vi "PH_Stepmotor_BaseClass.PC Set Axis Information.vi"(0 "i ref in":refnum<vi>, 1 "axis":i32=-1, 3 "Current Position (Steps)":i32, 4 "Axis Activity":T1, 5 "error in (no error)":errorcluster) -> (14 "i ref out":refnum<vi>, 19 "error out":errorcluster)   [LabVIEW 2014, in "PH_Stepmotor_BaseClass.lvlib"]
doc: "This VI stores in case of a change relevant information to own attributes and updates related DIM services."
uses:
  PH_Stepmotor_BaseClass.lvlib
  PH_Stepmotor_BaseClass.Axis Activity.ctl
  PH_Stepmotor_BaseClass.Axis Information.ctl
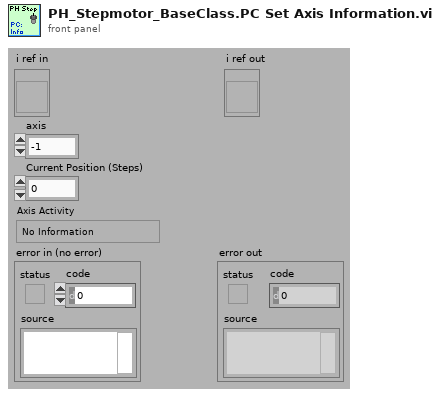
[diagram p1: front panel]
types:
  T1 = typedef "PH_Stepmotor_BaseClass.lvlib/PH_Stepmotor_BaseClass.Axis Activity.ctl" = enum16{"No Information", "stopped", "running", "Failure", "Alarm", "stopped at backward ES", "stopped at foreward ES"}
  T2 = typedef "PH_Stepmotor_BaseClass.lvlib/PH_Stepmotor_BaseClass.Axis Attributes.ctl" = cluster{"Settings":T3, "Endswitch?":bool, "DIM Service IDs":T5, "Activity":T1, "Configured?":bool, "Position":cluster{"Current":i32, "Target":i32}, "Position to set":cluster{"New?":bool, "Wanted":i32}, "Stop?":bool, "Reset?":bool, "Move?":bool, "Nothing connected?":bool}
  T3 = typedef "PH_Stepmotor_BaseClass.lvlib/PH_Stepmotor_BaseClass.Axis Settings.ctl" = cluster{"Sign change":bool, "Width":dbl, "Calibration":dbl, "Unit":string, "Motor Type":T4, "Unit Width":string, "Unit CF":string}
  T4 = typedef "PH_Stepmotor_BaseClass.lvlib/PH_Stepmotor_BaseClass.Motor Type.ctl" = enum16{"Unspecific", "OWIS 49.120.2633", "OWIS 49.060.1033", "OWIS 43.040.2558", "Diamond Motion 2200 series", "OWIS 49.120.266B.MV6", "Calorimeter", "Linear Stage 1", "MICOS VT-80", "MICOS VT-80 S", "Standa Rotstage nt0.95A", "PUF RA 320.200", "PUF RA 800.200", "PUF RA 800.400", "PUF RA 400.50", "1324.nn.800.50", "1324.n9c.800.50", "1324.nn.320.200", "1324.nn.400.200", "1324.nn.800.200", "1324.nn.400.50", "1324.8c9c.800.50", "1324.8c9c.400.200"}
  T5 = typedef "PH_Stepmotor_BaseClass.lvlib/PH_Stepmotor_BaseClass.Axis DIM Service IDs.ctl" = cluster{"Settings":i32, "Information":i32}
  T6 = typedef "PH_Stepmotor_BaseClass.lvlib/PH_Stepmotor_BaseClass.Axis Information.ctl" = cluster{"Scaled Position":dbl, "Activity":T1}
  T7 = typedef "PH_Stepmotor_BaseClass.lvlib/PH_Stepmotor_BaseClass.i attribute.ctl" = cluster{"Device Error":errorcluster, "Axes PSDB Thread":cluster{"Ref":refnum<vi>, "Q-Ref":refnum<queue>, "Data Status":T8}, "Axes":T2[], "Axes PSDB Infos":cluster{"GUI Name":string, "PSDB Instance ID":i32, "PSDB Status Service ID":i32, "Axis":i32, "Class":string}[], "GUI Refs":T9}
  T8 = typedef "PH_PSDBWriter.lvlib/PH_PSDBWriter.Data Status.ctl" = i16
  T9 = typedef "PH_Stepmotor_BaseClass.lvlib/PH_Stepmotor_BaseClass.GUI Refs.ctl" = cluster{"Axes Configuration":refnum<vi>, "Device Error":refnum<vi>, "Axes PSDB Infos":refnum<vi>}
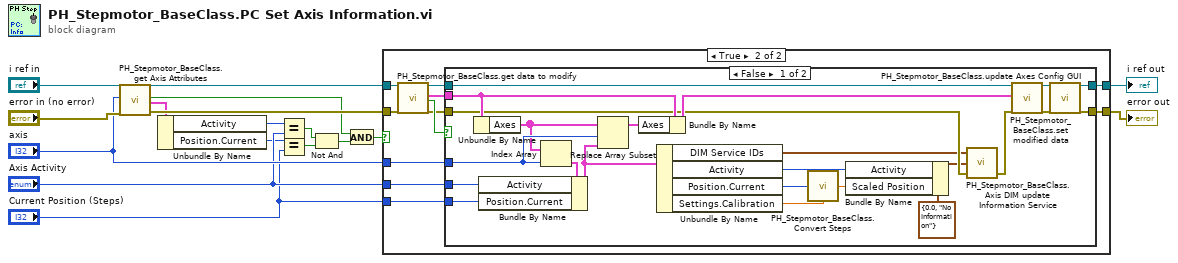
[diagram p0: block diagram]
diagram:
  n1 = call "PH_Stepmotor_BaseClass.get Axis Attributes.vi"("VI in"="i ref in", "Axis"="axis", "error in (no error)"="error in (no error)") -> ("VI out"=w12:refnum<vi>, "Axis found?"=w7:bool, "Axis Attributes"=w10:T2, "error out"=w14:errorcluster)  [unwired: 13 in]
  n2 = Unbundle By Name(w10) -> ("Activity"=w9:T1, "Position.Current"=w5:i32)
  n3 = Equal?(x=w9, y="Axis Activity") -> (x = y?=w3:bool)
  n4 = Equal?(x=w5, y="Current Position (Steps)") -> (x = y?=w2:bool)
  n5 = Not And(1:w2, 2:w3) -> (0:w1:bool)
  n6 = And(x=w7, y=w1) -> (x .and. y?=w8:bool)
  n7 = case shown="True" w8 {
    tunnel: [w19 w26] -> w16
    tunnel: [w18 w25] -> w15
    tunnel: w14 -> [w18 w24]
    tunnel: w12 -> [w19 w23]
    tunnel: "axis" -> [_ w22]
    tunnel: "Current Position (Steps)" -> [_ w21]
    tunnel: "Axis Activity" -> [_ w20]
    frame False {
    }
    frame True {
      n8 = call "PH_Stepmotor_BaseClass.get data to modify.vi"("i ref in"=w23, "error in (no error)"=w24) -> ("i ref out"=w28:refnum<vi>, "i attribute"=w27:T7, "timed out"=w30:bool, "error out"=w29:errorcluster)  [unwired: 14 in]
      n9 = case shown="False" w30 {
        tunnel: [w33 w55] -> w25
        tunnel: w29 -> [w43 w55]
        tunnel: [w31 w54] -> w26
        tunnel: w28 -> [w49 w54]
        tunnel: w27 -> [w52 _]
        tunnel: w22 -> [w48 _]
        tunnel: w21 -> [w45 _]
        tunnel: w20 -> [w44 _]
        frame False {
          n10 = Unbundle By Name(w52) -> ("Axes"=w47:T2[])
          n11 = Index Array(array=w47, index=w48) -> (element=w46:T2)
          n12 = Bundle By Name(cluster=w46, "Activity"=w44, "Position.Current"=w45) -> (w41:T2)
          n13 = Replace Array Subset(array=w47, new element=w41, index=w48) -> (w50:T2[])
          n14 = Bundle By Name(cluster=w52, "Axes"=w50) -> (w51:T7)
          n15 = Unbundle By Name(w41) -> ("DIM Service IDs"=w34:T5, "Activity"=w35:T1, "Position.Current"=w40:i32, "Settings.Calibration"=w36:dbl)
          n16 = call "PH_Stepmotor_BaseClass.Convert Steps.vi"("Postion (steps)"=w40, "Calibration Factor"=w36) -> ("Scaled Position"=w37:dbl)
          n17 = Bundle By Name(cluster=T6 {"Scaled Position"=0.0, "Activity"=enum."No Information"} ("Axis Information"), "Activity"=w35, "Scaled Position"=w37) -> (w38:T6)
          n18 = call "PH_Stepmotor_BaseClass.Axis DIM update Information Service.vi"("error in (no error)"=w43, "Axis Information"=w38, "Axis DIM IDs"=w34) -> ("error out"=w42:errorcluster)  [unwired: 2 in]
          n19 = call "PH_Stepmotor_BaseClass.set modified data.vi"("i ref in"=w49, "i attribute"=w51, "error in (no error)"=w42) -> ("i ref out"=w32:refnum<vi>, "error out"=w53:errorcluster)  [unwired: 15 in]
          n20 = call "PH_Stepmotor_BaseClass.update Axes Config GUI.vi"("VI in"=w32, "error in (no error)"=w53) -> ("VI out"=w31:refnum<vi>, "error out"=w33:errorcluster)  [unwired: 16 in]
        }
        frame True {
          (unwired) TRUE
        }
      }
    }
  }
  "error out" <- w15
  "i ref out" <- w16
